vi "Insight_Laser_Open.vi"(6 "Interface Type":enum16{"Ethernet", "Serial"}(ring), 7 "remote port or service name":u16=22141, 8 "error in (no error)":errorcluster, 10 "VISA resource name":refnum<visa-resource-name>, 11 "address":string="192.168.1.60") -> (0 "error out":errorcluster, 1 "*IDN?":string, 2 "VISA resource out":refnum<visa-resource-name>, 3 "connection ID out":refnum<k5>)   [LabVIEW 2010]
doc: "Insight Photonic Solutions\n\nThis VI performs read-write operations to-from the Insight Laser. The VI supports either Serial or TCP/IP connections.\n\nver 1.0 - original release"
uses:
  <vilib>/Instr/_visa.llb/VISA Configure Serial Port (Instr).vi
panel:
  out "Telnet Information":T1
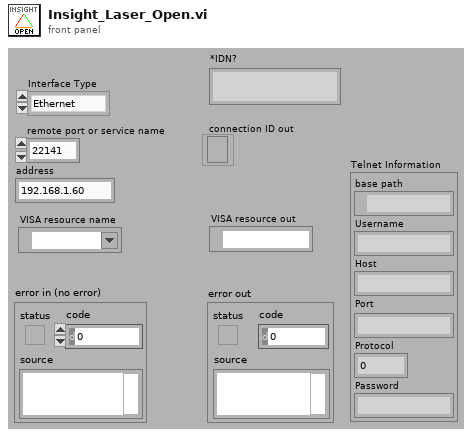
[diagram p1: front panel]
types:
  T1 = cluster{"base path":path, "Username":string, "Host":string, "Port":string, "Protocol":u16, "Password":string}
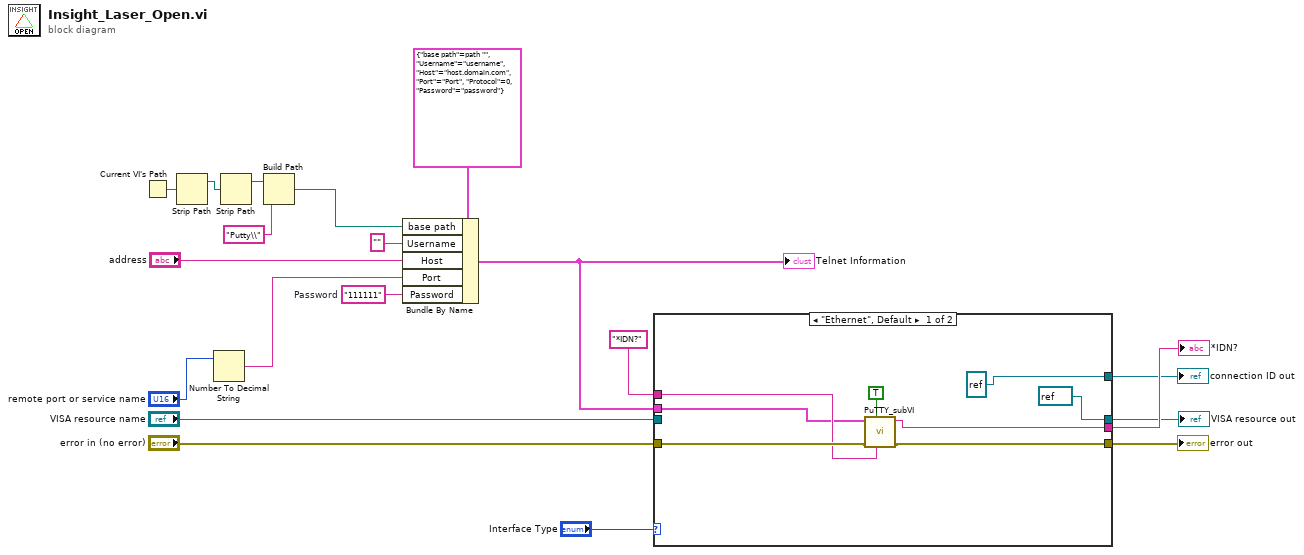
[diagram p0: block diagram]
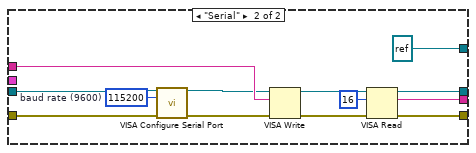
[diagram p2: hidden frame]
diagram:
  w8 = "111111"  # Password
  n1 = Current VI's Path() -> (path=w11:path)
  n2 = Strip Path(path=w11) -> (stripped path=w5:path)  [unwired: 1 out]
  n3 = Number To Decimal String(number="remote port or service name") -> (decimal integer string=w1:string)  [unwired: 1 in]
  n4 = Strip Path(path=w5) -> (stripped path=w6:path)  [unwired: 1 out]
  n5 = Build Path(base path=w6, name or relative path="Putty\\") -> (appended path=w9:path)
  n6 = Bundle By Name(cluster=T1 {"base path"=path "", "Username"="username", "Host"="host.domain.com", "Port"="Port", "Protocol"=0, "Password"="password"} ("PuTTY information"), "base path"=w9, "Username"="", "Host"="address", "Port"=w1, "Password"=w8) -> (w12:T1)
  "Telnet Information" <- w12
  n7 = case shown="\"Ethernet\", Default" "Interface Type" {
    tunnel: [w27 w39] -> w17
    tunnel: [refnum<visa-resource-name> refnum ("VISA resource name out") w38] -> w19
    tunnel: [w23 w37] -> w20
    tunnel: "VISA resource name" -> [_ w32]
    tunnel: "error in (no error)" -> [w26 w34]
    tunnel: "*IDN?" ("String") -> [w24 w36]
    tunnel: [refnum<k5> refnum ("connection ID") refnum<k5> refnum ("connection ID")] -> w14
    tunnel: w12 -> [w21 _]
    frame "Ethernet", Default {
      n8 = call "PuTTY_subVI.vi"("Command(s) to Execute"=w24, "Hide DOS\nWindow?"=TRUE ("Hide DOS\nWindow?"), "error in"=w26, "PuTTY information"=w21) -> ("error out"=w27:errorcluster, "Command Return Value(s)"=w23:string)  [unwired: 5 in, 1 out]
    }
    frame "Serial" {
      w30 = u32 115200  # baud rate (9600)
      n9 = call-poly "VISA Configure Serial Port"("VISA resource name"=w32, "baud rate (9600)"=w30, "error in (no error)"=w34) -> ("VISA resource name out"=w31:refnum<visa-resource-name>, "error out"=w33:errorcluster)  [unwired: 11 in]
      n10 = VISA Write(VISA resource name=w31, write buffer=w36, error in (no error)=w33) -> (VISA resource name out=w40:refnum<visa-resource-name>, error out=w41:errorcluster)  [unwired: 1 out]
      n11 = VISA Read(VISA resource name=w40, byte count=u32 16, error in (no error)=w41) -> (VISA resource name out=w38:refnum<visa-resource-name>, read buffer=w37:string, error out=w39:errorcluster)  [unwired: 1 out]
    }
  }
  "error out" <- w17
  "VISA resource out" <- w19
  "*IDN?" <- w20
  "connection ID out" <- w14
